vi "Order Custom Device Channel Value Table.vi"(9 "Values":dbl[](array[numeric])=[1.0, 2.0, 3.0, 4.0, 5.0, 0.0], 10 "Names":string[](array[string])=["Cat", "Dog", "Chicken", "Snake", "Zebra", "Mouse"]) -> (2 "Names (Ordered)":string[](array[string]))   [LabVIEW 2019, in "Profile Interpolation Shared.lvlib"]
uses:
  Profile Interpolation Shared.lvlib
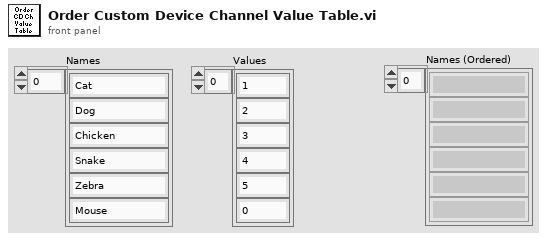
[diagram p1: front panel]
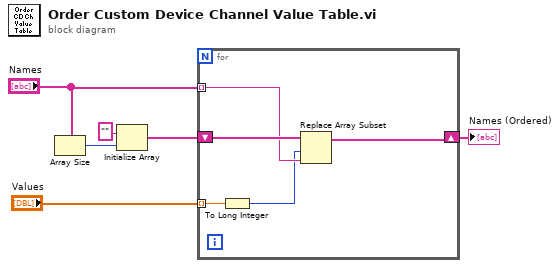
[diagram p0: block diagram]
diagram:
  n1 = Array Size(array="Names") -> (size(s)=w4:i32)
  n2 = Initialize Array("", w4) -> (w2:string[])
  n3 = for {
    tunnel: "Names" -> [w10] mode=indexing
    tunnel: "Values" -> [w9] mode=indexing
    shift-right: [w7] -> w1
    shift-left: w2 -> [w11]
    n4 = To Long Integer(number=w9) -> (32bit integer=w8:i32)
    n5 = Replace Array Subset(array=w11, new element=w10, index=w8) -> (w7:string[])
  }
  "Names (Ordered)" <- w1
